vi "Get Package Attribute Value.vi"(8 "error in (no error)":errorcluster, 9 "package attribute":string, 10 "package name":string, 11 "NI Package Builder solution (.pbs)":path) -> (0 "error out":errorcluster, 1 "Value":string, 2 "package name out":string, 3 "NI Package Builder solution out":path)   [LabVIEW 2017, in "NIPB Solution API.lvlib"]
doc: "Gets the value of the specified attribute of the specified package in the specified NI Package Builder solution (.pbs).\n\nIf the <b>package name</b> input is unwired, this VI will perform this operation on the first package in the NI Package Builder solution and output the corresponding package name in the <b>package name out</b> output."
uses:
  NIPB Solution API.lvlib
  <resource>/objmgr/DOMUserDefRef.rc
  <vilib>/xml/NI_XML.lvlib
  <vilib>/xml/Load XML File.vi
  <vilib>/xml/Close Reference(Node).vi
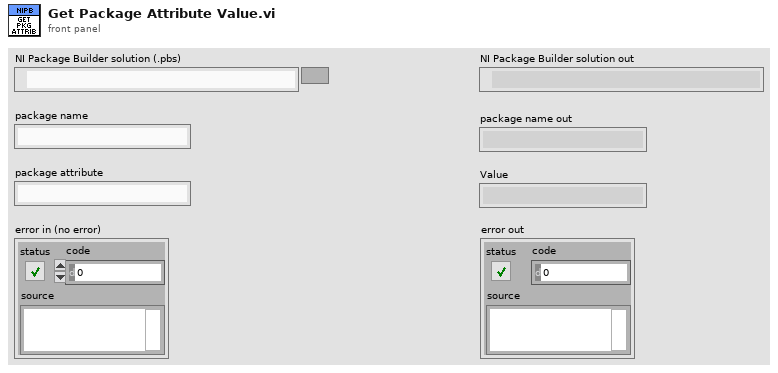
[diagram p1: front panel]
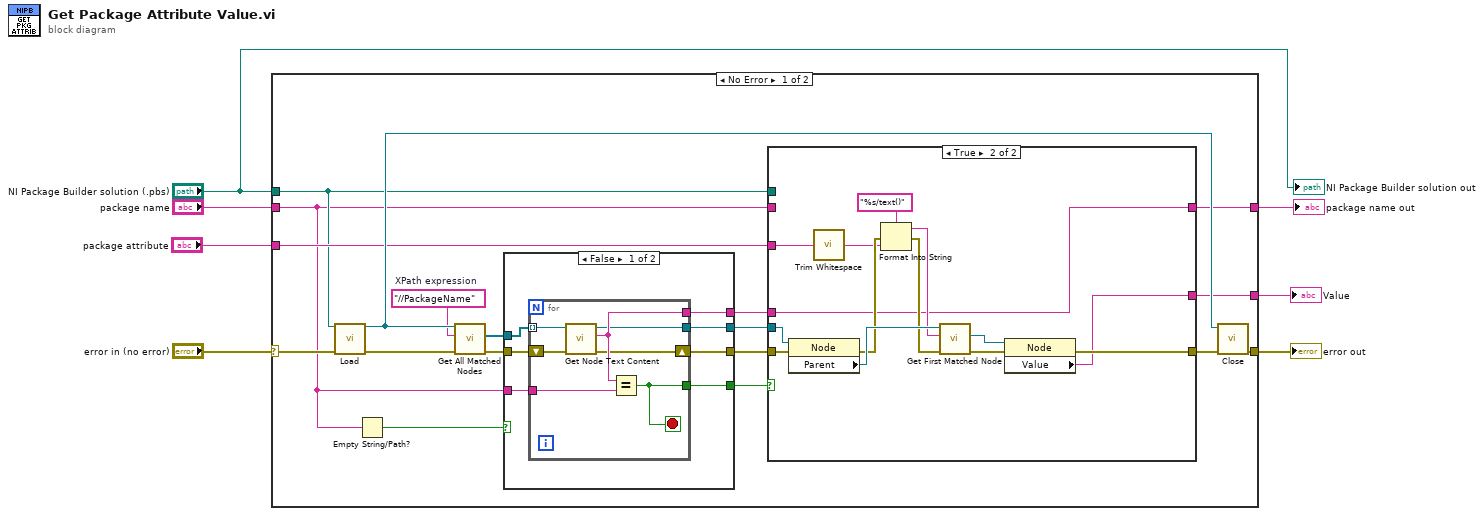
[diagram p0: block diagram]
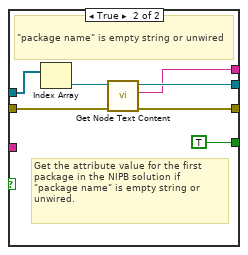
[diagram p2: hidden frame]
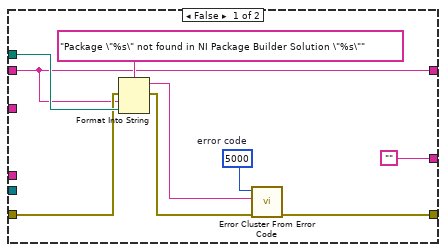
[diagram p3: hidden frame]
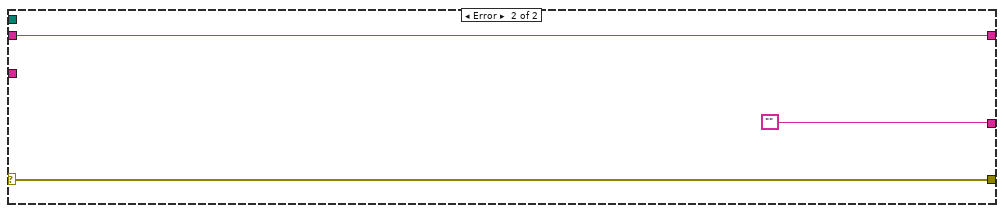
[diagram p4: hidden frame]
diagram:
  n1 = case shown="No Error" "error in (no error)" {
    selector: "error in (no error)" -> [w13 w72]
    tunnel: [w24 w72] -> w7
    tunnel: "package attribute" -> [w23 _]
    tunnel: [w22 ""] -> w5
    tunnel: "package name" -> [w11 w70]
    tunnel: "NI Package Builder solution (.pbs)" -> [w12 _]
    tunnel: [w9 w70] -> w1
    frame No Error {
      w15 = "//PackageName"  # XPath expression
      n2 = call-poly <vilib>:"Load.vi"("path to XML document"=w12, "error in (no error)"=w13) -> ("DOM document out"=w25:refnum<k20>, "error out"=w14:errorcluster)  [unwired: 11 in, 1 out]
      n3 = Empty String/Path?(string/path=w11) -> (empty?=w10:bool)
      n4 = call <vilib>:"Get All Matched Nodes.vi"("error in (no error)"=w14, "XPath expression"=w15, "node in"=w25) -> ("error out"=w17:errorcluster, "node result array"=w16:refnum<k20>[])  [unwired: 6 in, 1 out]
      n5 = case shown="False" w10 {
        tunnel: w11 -> [w32 _]
        tunnel: [w31 w43] -> w20
        tunnel: [w30 w41] -> w19
        tunnel: [w29 TRUE] -> w18
        tunnel: w17 -> [w28 w44]
        tunnel: w16 -> [w27 w46]
        tunnel: [w26 w40] -> w8
        frame False {
          n6 = for {
            tunnel: w27 -> [w36] mode=indexing
            tunnel: [w39] -> w26
            tunnel: w32 -> [w38]
            tunnel: [w37] -> w29
            tunnel: [w33] -> w30
            shift-right: [w34] -> w31
            shift-left: w28 -> [w35]
            stop <- w37 stop-if-true
            n7 = call <vilib>:"Get Node Text Content.vi"("error in (no error)"=w35, "node in"=w36) -> ("error out"=w34:errorcluster, "node text"=w39:string, "node out"=w33:refnum<k20>)  [unwired: 7 in]
            n8 = Equal?(x=w39, y=w38) -> (x = y?=w37:bool)
          }
        }
        frame True {
          # "Get the attribute value for the first package in the NIPB solution if \"package name\" is empty string or unwired."
          # "\"package name\" is empty string or unwired"
          n9 = Index Array(array=w46) -> (element=w42:refnum<k20>)  [unwired: 1 in]
          n10 = call <vilib>:"Get Node Text Content.vi"("error in (no error)"=w44, "node in"=w42) -> ("error out"=w43:errorcluster, "node text"=w40:string, "node out"=w41:refnum<k20>)  [unwired: 7 in]
        }
      }
      n11 = case shown="True" w18 {
        tunnel: w19 -> [_ w69]
        tunnel: w20 -> [w51 w68]
        tunnel: w12 -> [w52 _]
        tunnel: [w55 w64] -> w21
        tunnel: w11 -> [w47 _]
        tunnel: ["" w63] -> w22
        tunnel: w23 -> [_ w62]
        tunnel: [w47 w56] -> w9
        tunnel: w8 -> [_ w56]
        frame False {
          w54 = 5000  # error code
          n12 = Format Into String(format string="Package \"%s\" not found in NI Package Builder Solution \"%s\"", error in=w51, w47, w52) -> (resulting string=w49:string, error out=w50:errorcluster)  [unwired: 1 in]
          n13 = call <vilib>:"Error Cluster From Error Code.vi"("error in (no error)"=w50, "error message (\"\")"=w49, "error code (0)"=w54) -> ("error out"=w55:errorcluster)  [unwired: 6 in]
        }
        frame True {
          n14 = property class="Node"(reference=w69, error in=w68) -> (error out=w59:errorcluster, "Parent"=w65:refnum<k20>)  [unwired: 1 out]
          n15 = call <vilib>:"Trim Whitespace.vi"("string"=w62) -> ("trimmed string"=w57:string)  [unwired: 1 in]
          n16 = Format Into String(format string="%s/text()", error in=w59, w57) -> (resulting string=w60:string, error out=w58:errorcluster)  [unwired: 1 in]
          n17 = call <vilib>:"Get First Matched Node.vi"("error in (no error)"=w58, "XPath expression"=w60, "node in"=w65) -> ("error out"=w66:errorcluster, "node result"=w67:refnum<k20>)  [unwired: 6 in, 1 out]
          n18 = property class="Node"(reference=w67, error in=w66) -> (error out=w64:errorcluster, "Value"=w63:string)  [unwired: 1 out]
        }
      }
      n19 = call-poly <vilib>:"Close.vi"("error in (no error)"=w21, "node"=w25) -> ("error out"=w24:errorcluster)  [unwired: 7 in]
    }
    frame Error {
    }
  }
  "error out" <- w7
  "Value" <- w5
  "package name out" <- w1
  "NI Package Builder solution out" <- "NI Package Builder solution (.pbs)"
